vi "Calculated Shooter Speed.vi"() -> ()   [LabVIEW 2012]
panel:
  in  "Calculated Shooter Speed":dbl
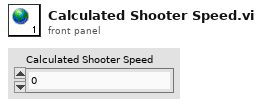
[diagram p1: front panel]
diagram:
